vi "init.keithley.vi"() -> ()   [LabVIEW 2020]
panel:
  out "data":string
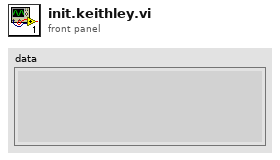
[diagram p1: front panel]
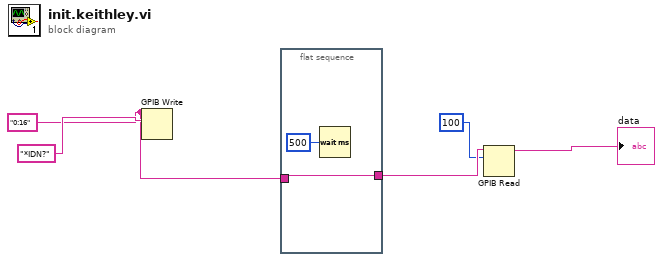
[diagram p0: block diagram]
diagram:
  w4 = "0:16"
  n1 = GPIB Write(0:w4, 1:"*IDN?") -> ()  [unwired: 3 in, 2 out]
  n2 = flat-sequence {
    tunnel: w4 -> [w6]
    tunnel: [w6] -> w3
    frame #0 {
      n3 = Wait (ms)(milliseconds to wait=u32 500) -> ()  [unwired: 1 out]
    }
  }
  n4 = GPIB Read(0:w3, 1:100 ("byte count")) -> (5:→"data":string)  [unwired: 3 in, 2 out]
